vi "Set Baud Rate.vi"(8 "error in":errorcluster, 10 "Baud Rate":T1(ring), 11 "PCAN in":refnum<class "PCAN.lvclass">) -> (0 "error out":errorcluster, 3 "PCAN out":refnum<class "PCAN.lvclass">)   [LabVIEW 2023, in "PCAN.lvclass"]
uses:
  PCAN.lvclass
  PCAN.lvclass/PCAN.ctl
  Configurations/CFG Base/CFG Base.lvclass
  44f1022e-da92-44a8-9875-745310e8b83f.vi
  <instrlib>/KDI Digital Instrumentation/API_for_PCAN_BASIC_FD/TPCANBaudrate.ctl
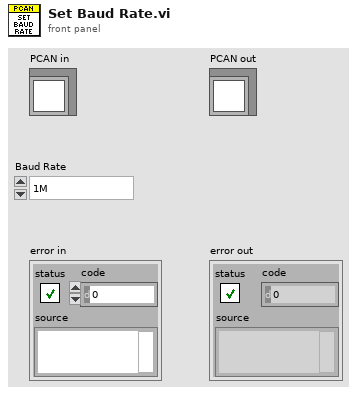
[diagram p1: front panel]
types:
  T1 = enum16{"1M", "800k", "500k", "250k", "125k", "50k", "25k", "10k"}
  T2 = typedef "TPCANBaudrate.ctl" = enum16{"PCAN_BAUD_1M 0x0014", "PCAN_BAUD_800K 0x0016", "PCAN_BAUD_500K 0x001C", "PCAN_BAUD_250K 0x011C", "PCAN_BAUD_125K 0x031C", "PCAN_BAUD_100K 0x432F", "PCAN_BAUD_95K 0xC34E", "PCAN_BAUD_83K 0x852B", "PCAN_BAUD_50K 0x472F", "PCAN_BAUD_47K 0x1414", "PCAN_BAUD_33K 0x8B2F", "PCAN_BAUD_20K 0x532F", "PCAN_BAUD_10K 0x672F", "PCAN_BAUD_5K 0x7F7F", "User Baudrate"}
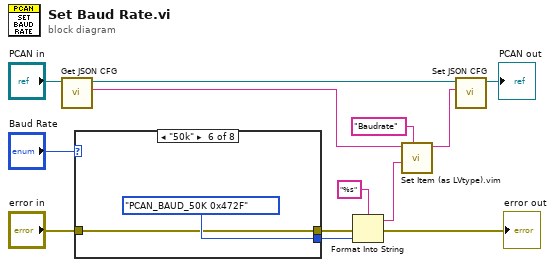
[diagram p0: block diagram]
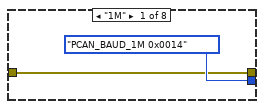
[diagram p2: hidden frame]
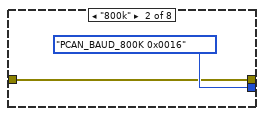
[diagram p3: hidden frame]
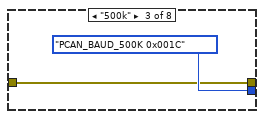
[diagram p4: hidden frame]
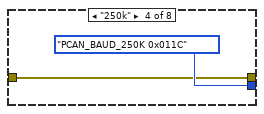
[diagram p5: hidden frame]
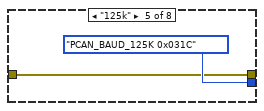
[diagram p6: hidden frame]
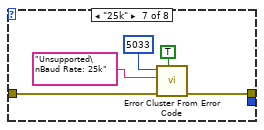
[diagram p7: hidden frame]
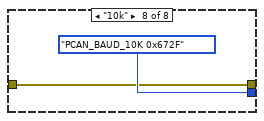
[diagram p8: hidden frame]
diagram:
  n1 = call "Get JSON CFG.vi"("CFG Base in"="PCAN in") -> ("<JSON>CFG"=w11:string, "CFG Base out"=w12:refnum<class "PCAN.lvclass">)  [unwired: 9 in]
  n2 = case shown="\"50k\"" "Baud Rate" {
    tunnel: [TPCANBaudrate."PCAN_BAUD_1M 0x0014" ("TPCANBaudrate") TPCANBaudrate."PCAN_BAUD_800K 0x0016" ("TPCANBaudrate") TPCANBaudrate."PCAN_BAUD_500K 0x001C" ("TPCANBaudrate") TPCANBaudrate."PCAN_BAUD_250K 0x011C" ("TPCANBaudrate") TPCANBaudrate."PCAN_BAUD_125K 0x031C" ("TPCANBaudrate") TPCANBaudrate."PCAN_BAUD_50K 0x472F" ("TPCANBaudrate") _ TPCANBaudrate."PCAN_BAUD_10K 0x672F" ("TPCANBaudrate")] -> w7
    tunnel: "error in" -> [w14 w16 w18 w20 w22 w24 w30 w31]
    tunnel: [w14 w16 w18 w20 w22 w24 w29 w31] -> w1
    frame "1M" {
    }
    frame "800k" {
    }
    frame "500k" {
    }
    frame "250k" {
    }
    frame "125k" {
    }
    frame "50k" {
    }
    frame "25k" {
      n3 = call <vilib>:"Error Cluster From Error Code.vi"("show call chain? (False)"=TRUE, "error in (no error)"=w30, "error message (\"\")"="Unsupported\nBaud Rate: 25k" ("error message (\"\")"), "error code (0)"=5033) -> ("error out"=w29:errorcluster)  [unwired: 5 in]
    }
    frame "10k" {
    }
  }
  n4 = Format Into String(format string="%s", error in=w1, w7) -> (resulting string=w6:string, error out=→"error out":errorcluster)  [unwired: 1 in]
  n5 = call "Set Item (as LVtype).vim"("$Path or Item Name"="Baudrate", "Anything"=w6, "JSON"=w11) -> ("<JSON>"=w3:string)  [unwired: 5 in, 2 out]
  n6 = call "Set JSON CFG.vi"("<JSON>CFG"=w3, "CFG Base in"=w12) -> ("CFG Base out"=→"PCAN out":refnum<class "PCAN.lvclass">)  [unwired: 9 in]
